vi "U8_To_Bin.vi"(10 "U16[]":u16[](array[numeric]) format="%.0x") -> (2 "Bit[]":u8[](array[numeric]))   [LabVIEW 2017]
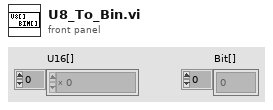
[diagram p1: front panel]
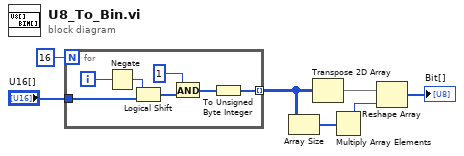
[diagram p0: block diagram]
diagram:
  n1 = for {
    N: 16 -> [_]
    tunnel: "U16[]" -> [w14]
    tunnel: [w8] -> w5 mode=indexing
    i -> [w13]
    n2 = Negate(x=w13) -> (-x=w12:i32)
    n3 = Logical Shift(y=w12, x=w14) -> (x << y=w11:u16[])
    n4 = And(x=u16 1, y=w11) -> (x .and. y?=w9:u16[])
    n5 = To Unsigned Byte Integer(number=w9) -> (unsigned 8bit integer=w8:u8[])
  }
  n6 = Array Size(array=w5) -> (size(s)=w6:i32[])
  n7 = Transpose 2D Array(2D array=w5) -> (transposed array=w1:u8[][])
  n8 = Multiply Array Elements(1:w6) -> (0:w4:i32)
  n9 = Reshape Array(w1, w4) -> (→"Bit[]":u8[])
